vi "(SubVI) Create AxisPI.vi"(4 "axis":u32) -> (0 "Axis String":string, 1 "Axis String Array":string[](array[string]), 2 "Axis Array":i32[](array[numeric]))   [LabVIEW 2014]
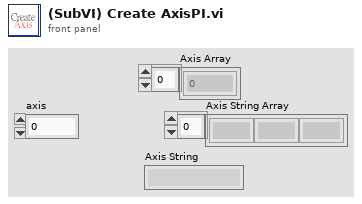
[diagram p1: front panel]
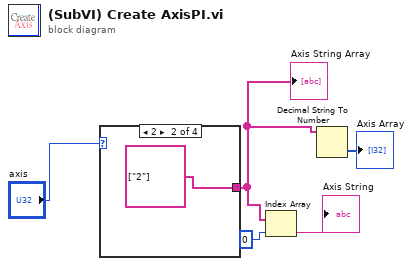
[diagram p0: block diagram]
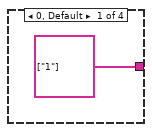
[diagram p2: hidden frame]
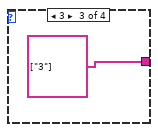
[diagram p3: hidden frame]
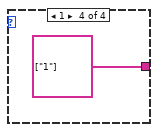
[diagram p4: hidden frame]
diagram:
  n1 = case shown="2" "axis" {
    tunnel: [string[] ["1"] string[] ["2"] string[] ["3"] string[] ["1"]] -> w2
    frame 0, Default {
    }
    frame 2 {
    }
    frame 3 {
    }
    frame 1 {
    }
  }
  "Axis String Array" <- w2
  n2 = Index Array(array=w2, index=0) -> (element=→"Axis String":string)
  n3 = Decimal String To Number(string=w2) -> (number=→"Axis Array":i32[])  [unwired: 3 out]
